vi "更新程序.vi"() -> ()   [LabVIEW 2016, in "数据传输系统.lvlib"]
uses:
  <vilib>/Utility/config.llb/Read Key (String).vi
  <vilib>/Utility/config.llb/Read Key (I32).vi
  <vilib>/Utility/config.llb/NI_LVConfig.lvlib
panel:
  out "软件版本 2":string caption="目标软件版本"
  out "软件版本":string caption="当前软件版本"
  out "下载的文件名":string
  out "目标文件夹名":string
  out "waittime":u8
  out "端口号":i32
  out "IP地址":string
  out "步骤":string
  out "枚举":T1(ring)
  in  "目标路径（使用对话框）":path
  out "下载保存目录":path
  out "更新进度":u8(slide) scale=0.0..100.0
  # "1.先下载更新-------2.关闭主应用-------3.替换应用--------4.打开主应用-----------5.关闭本程序"
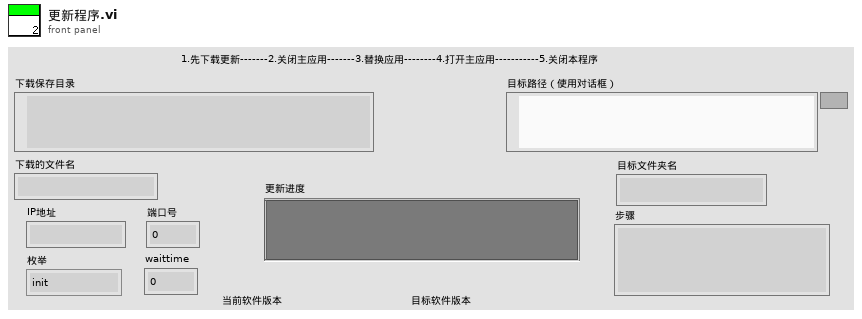
[diagram p1: front panel]
types:
  T1 = enum16{"init", "download", "close", "replace", "open", "over"}
  T2 = enum16{"open", "replace", "create", "open or create", "replace or create", "replace or create with confirmation"}
  T3 = cluster{"网络灯":bool, "接收中":bool, "已接收百分比":u8, "接收成功次数":dbl, "当前步骤":enum16{"init", "receivehead", "receivecontent", "receivesuccess", "over"}, "文件名":string, "error out":errorcluster}
  T4 = typedef "NI_LVConfig.lvlib/Config Data RefNum.ctl" = refnum<k1>
  T5 = enum32{"Bad", "Idle", "Run top level", "Running"}
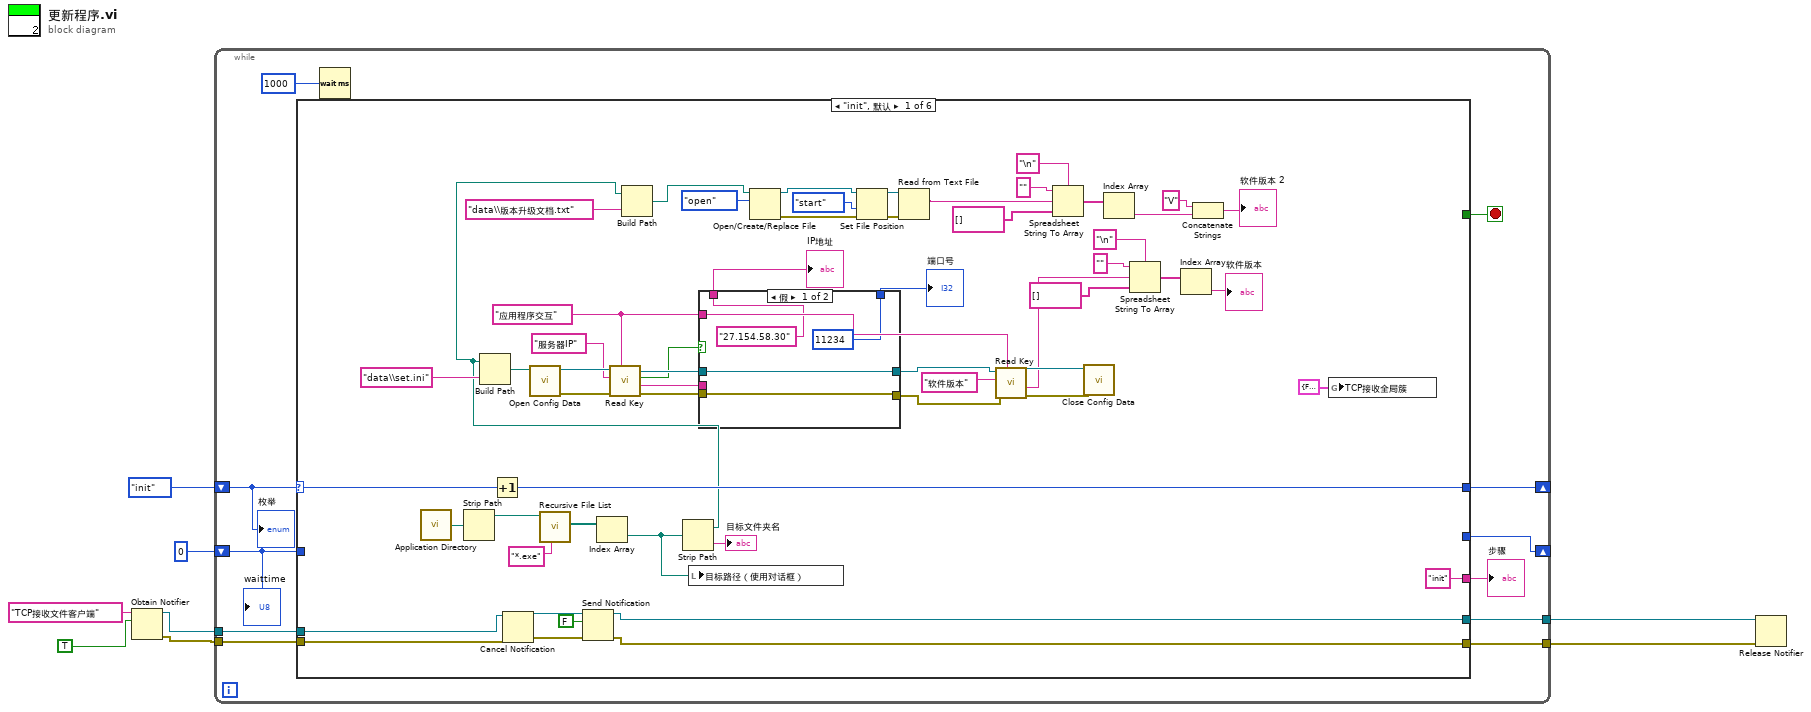
[diagram p0: block diagram]
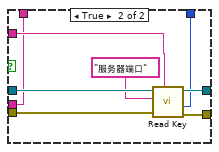
[diagram p2: hidden frame]
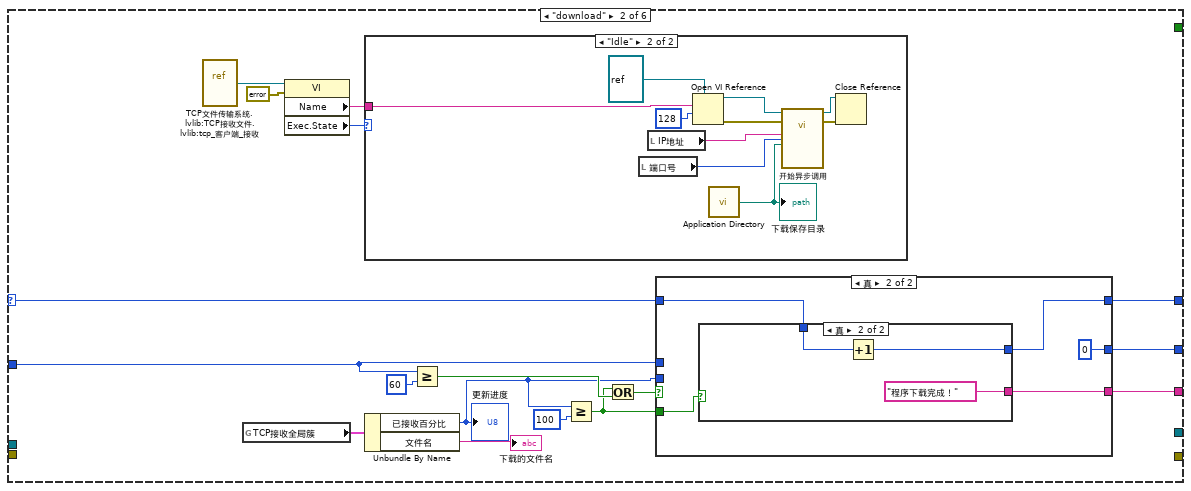
[diagram p3: hidden frame]
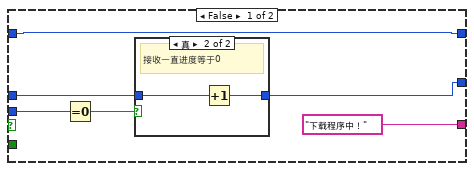
[diagram p5: hidden frame]
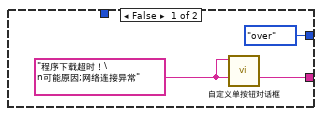
[diagram p7: hidden frame]
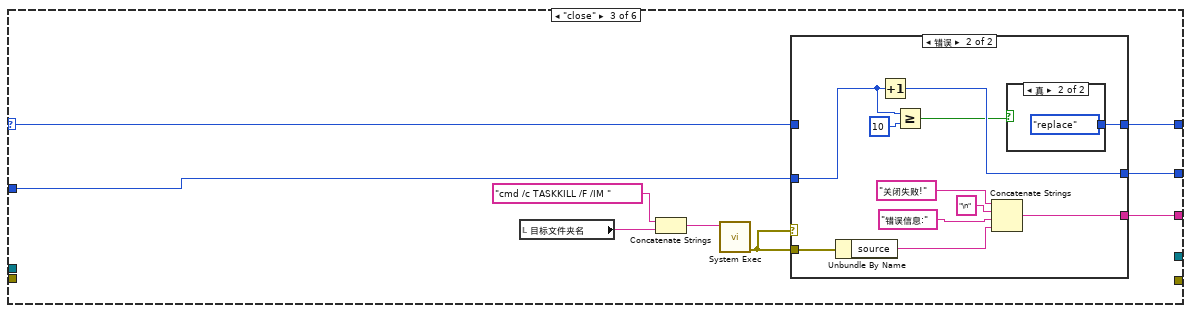
[diagram p8: hidden frame]
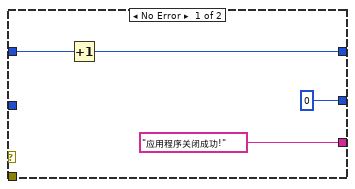
[diagram p9: hidden frame]
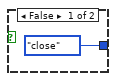
[diagram p10: hidden frame]
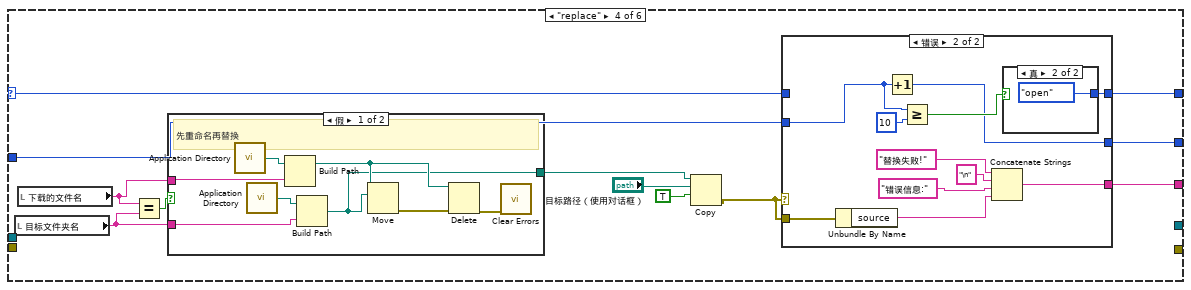
[diagram p11: hidden frame]
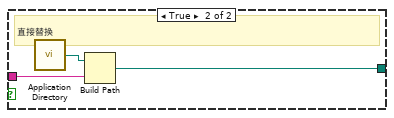
[diagram p12: hidden frame]
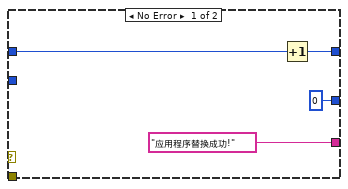
[diagram p13: hidden frame]
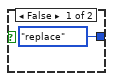
[diagram p14: hidden frame]
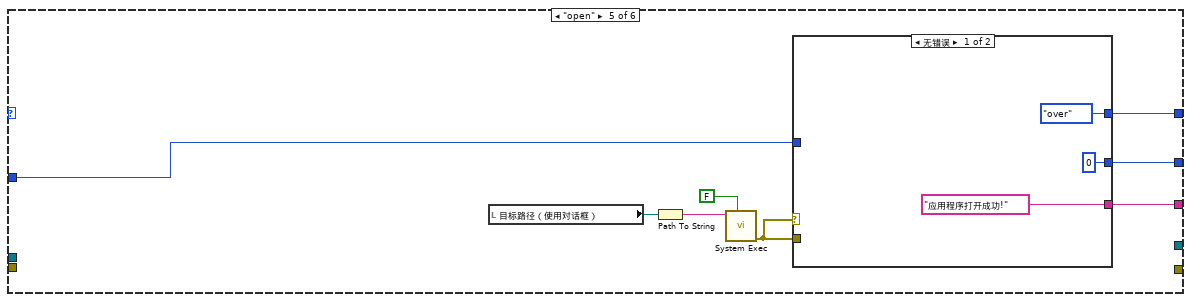
[diagram p15: hidden frame]
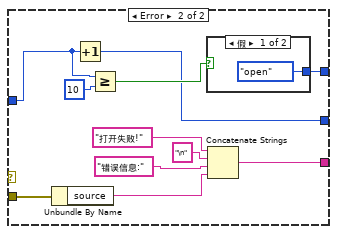
[diagram p16: hidden frame]
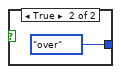
[diagram p17: hidden frame]
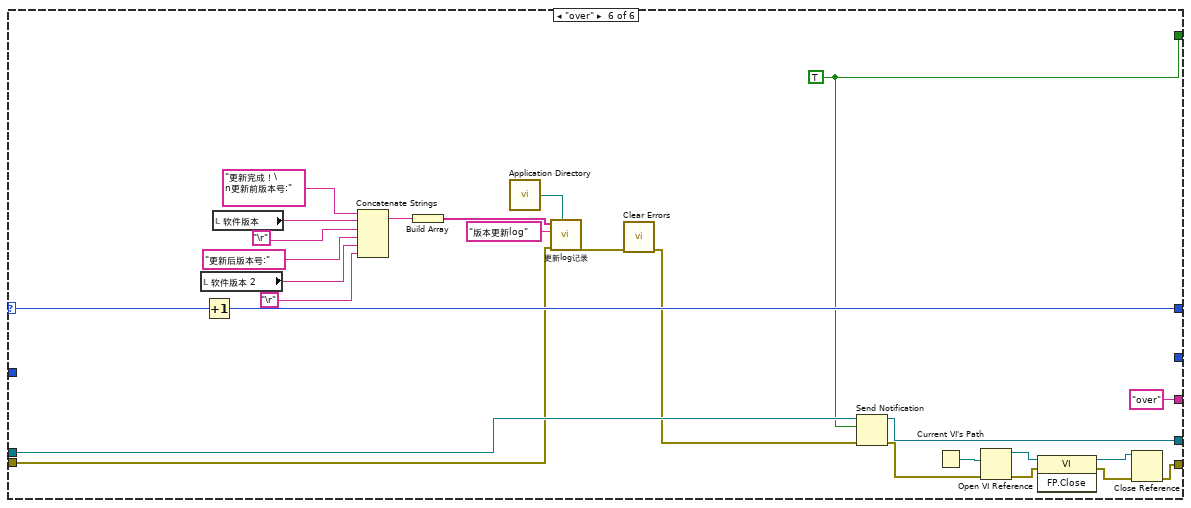
[diagram p18: hidden frame]
diagram:
  n1 = Obtain Notifier(name (unnamed)="TCP接收文件客户端" ("名称（未命名）"), notification data type=TRUE) -> (notifier out=w4:refnum<notifier>, error out=w3:errorcluster)  [unwired: 2 in, 1 out]
  n2 = while {
    shift-right: [w18] -> _
    shift-left: T1."init" -> [w19]
    shift-right: [w13] -> _
    shift-left: u8 0 ("y") -> [w14]
    tunnel: w4 -> [w12]
    tunnel: w3 -> [w11]
    tunnel: [w10] -> w2
    tunnel: [w9] -> w1
    stop <- w17 stop-if-true
    n3 = case shown="\"init\", 默认" w19 {
      selector: w19 -> [w76 w98 w140 w172 _ w250]
      tunnel: [w75 w99 w139 w171 w204 w249] -> w18
      tunnel: [_ _ _ _ _ w245] -> w17
      tunnel: ["init" ("步骤") w95 w138 w170 w203 "over" ("步骤")] -> w15
      tunnel: w14 -> [_ w97 w137 w169 w202 _]
      tunnel: [_ w104 w136 w168 w201 _] -> w13
      tunnel: w12 -> [w73 _ _ _ _ w247]
      tunnel: w11 -> [w72 _ _ _ _ w237]
      tunnel: [w68 _ _ _ _ w246] -> w10
      tunnel: [w67 _ _ _ _ w229] -> w9
      frame "init", Default {
        w47 = "应用程序交互" ("section")
        n4 = call <vilib>:"Application Directory.vi"() -> ("Application Directory"=w64:path)
        n5 = Strip Path(path=w64) -> (stripped path=w60:path)  [unwired: 1 out]
        n6 = Increment(x=w76) -> (x+1=w75:T1)
        n7 = Cancel Notification(0:w73, 3:w72) -> (8:w71:refnum<notifier>, 11:w69:errorcluster)  [unwired: 1 out]
        n8 = call <vilib>:"Recursive File List.vi"("pattern"="*.exe", "Folder Path"=w60) -> ("All Files in Dir"=w62:path[])  [unwired: 5 in, 4 out]
        n9 = Send Notification(notification=FALSE ("通知"), notifier=w71, error in (no error)=w69) -> (notifier out=w68:refnum<notifier>, error out=w67:errorcluster)
        n10 = Index Array(array=w62) -> (element=w65:path)  [unwired: 1 in]
        n11 = Strip Path(path=w65) -> (stripped path=w20:path, name=→"目标文件夹名":string)
        n12 = Build Path(base path=w20, name or relative path="data\\set.ini" ("名称或相对路径")) -> (appended path=w59:path)
        n13 = call <vilib>:"Open Config Data.vi"("configuration file path"=w59) -> ("error out"=w56:errorcluster, "refnum"=w57:T4)  [unwired: 8 in, 1 out]
        n14 = call-poly <vilib>:"Read Key.vi"("section"=w47, "error in (no error)"=w56, "key"="服务器IP" ("section"), "refnum"=w57) -> ("error out"=w46:errorcluster, "value"=w45:string, "found?"=w43:bool, "refnum out"=w55:T4)  [unwired: 4 in]
        n15 = Build Path(base path=w20, name or relative path="data\\版本升级文档.txt" ("名称或相对路径")) -> (appended path=w28:path)
        n16 = local write "目标路径（使用对话框）"(w65) -> ()
        n17 = case shown="假" w43 {
          tunnel: w55 -> [w78 w88]
          tunnel: w46 -> [w77 w87]
          tunnel: [w78 w85] -> w53
          tunnel: [w77 w84] -> w52
          tunnel: [11234 ("value") w83] -> w48
          tunnel: w47 -> [_ w82]
          tunnel: w45 -> [_ w81]
          tunnel: ["27.154.58.30" ("key") w81] -> w44
          frame False {
          }
          frame True {
            n18 = call-poly <vilib>:"Read Key.vi"("section"=w82, "error in (no error)"=w87, "key"="服务器端口" ("section"), "refnum"=w88) -> ("error out"=w84:errorcluster, "value"=w83:i32, "refnum out"=w85:T4)  [unwired: 4 in, 1 out]
          }
        }
        "IP地址" <- w44
        "端口号" <- w48
        n19 = Open/Create/Replace File(file path (use dialog)=w28, operation (0:open)=T2."open" ("操作(0:open)")) -> (refnum out=w23:refnum<file>, error out=w24:errorcluster)  [unwired: 4 in, 1 out]
        n20 = Set File Position(refnum=w23, from (0:start)=enum16{"start", "end", "current"}."start" ("自（0:起始）"), error in=w24) -> (refnum out=w27:refnum<file>, error out=w25:errorcluster)  [unwired: 1 in]
        n21 = Read from Text File(file (use dialog)=w27, error in=w25) -> (text=w35:string)  [unwired: 2 in, 3 out]
        n22 = call-poly <vilib>:"Read Key.vi"("section"=w47, "error in (no error)"=w52, "key"="软件版本", "refnum"=w53) -> ("error out"=w49:errorcluster, "value"=w37:string, "refnum out"=w50:T4)  [unwired: 4 in, 1 out]
        n23 = Spreadsheet String To Array(delimiter (Tab)="\n" ("分隔符(Tab)"), format string="" ("格式字符串"), spreadsheet string=w35, array type (2D Dbl)=string[] []) -> (array=w32:string[])
        n24 = call <vilib>:"Close Config Data.vi"("error in (no error)"=w49, "refnum"=w50) -> ()  [unwired: 8 in, 2 out]
        n25 = Index Array(array=w32) -> (element=w33:string)  [unwired: 1 in]
        n26 = Spreadsheet String To Array(delimiter (Tab)="\n" ("分隔符(Tab)"), format string="" ("格式字符串"), spreadsheet string=w37, array type (2D Dbl)=string[] []) -> (array=w39:string[])
        n27 = Index Array(array=w39) -> (element=→"软件版本":string)  [unwired: 1 in]
        n28 = Concatenate Strings("V" ("字符串"), w33) -> (→"软件版本 2":string)
        n29 = global write "全局变量1.vi" "TCP接收全局簇"(T3 {"网络灯"=FALSE, "接收中"=FALSE, "已接收百分比"=0, "接收成功次数"=0.0, "当前步骤"=enum."init", "文件名"="", "error out"={"status"=FALSE, "code"=0, "source"=""}} ("TCP接收全局簇")) -> ()
      }
      frame "download" {
        n30 = vi-ref "TCP文件传输系统.lvlib:TCP接收文件.lvlib:tcp_客户端_接收.vi"() -> (w90:refnum<vi>)
        n31 = global read "全局变量1.vi" "TCP接收全局簇"() -> (w96:T3)
        n32 = property class="VI"(reference=w90, error in=errorcluster {"status"=FALSE, "code"=0, "source"=""} ("错误输出")) -> ("Name"=w91:string, "Exec.State"=w93:T5)  [unwired: 2 out]
        n33 = case shown="\"Idle\"" w93 {
          tunnel: w91 -> [_ w114]
          frame "Bad", Default {
          }
          frame "Idle" {
            n34 = local read "端口号"() -> (w106:i32)
            n35 = local read "IP地址"() -> (w107:string)
            n36 = Open VI Reference(type specifier VI Refnum (for type only)=refnum<vi> refnum, vi path=w114, options=128 ("选项")) -> (vi reference=w112:refnum<vi>, error out=w110:errorcluster)  [unwired: 3 in]
            n37 = call <vilib>:"Application Directory.vi"() -> ("Application Directory"=w115:path)
            "下载保存目录" <- w115
            n38 = call-by-ref "开始异步调用"(reference=w112, error in=w110, "IP地址"=w107, "端口号"=w106, "储存路径"=w115) -> (reference out=w108:refnum<vi>, error out=w109:errorcluster)  [unwired: 17 in]
            n39 = Close Reference(reference=w108, error in (no error)=w109) -> ()  [unwired: 1 out]
          }
        }
        n40 = Unbundle By Name(w96) -> ("已接收百分比"=w100:u8, "文件名"=→"下载的文件名":string)
        "更新进度" <- w100
        n41 = Greater Or Equal?(x=w97, y=u8 60) -> (x >= y?=w102:bool)
        n42 = Greater Or Equal?(x=w100, y=u8 100) -> (x >= y?=w94:bool)
        n43 = Or(x=w94, y=w102) -> (x .or. y?=w101:bool)
        n44 = case shown="真" w101 {
          tunnel: w97 -> [w121 _]
          tunnel: [w120 u8 0] -> w104
          tunnel: w100 -> [w118 _]
          tunnel: [w117 w125] -> w99
          tunnel: w98 -> [w117 w126]
          tunnel: ["下载程序中！" w127] -> w95
          tunnel: w94 -> [_ w128]
          frame False {
            n45 = Equal To 0?(x=w118) -> (x = 0?=w119:bool)
            n46 = case shown="真" w119 {
              tunnel: w121 -> [w122 w124]
              tunnel: [w122 w123] -> w120
              frame False {
              }
              frame True {
                # "接收一直进度等于0"
                n47 = Increment(x=w124) -> (x+1=w123:u8)
              }
            }
          }
          frame True {
            n48 = case shown="真" w128 {
              tunnel: [w130 "程序下载完成！"] -> w127
              tunnel: w126 -> [_ w133]
              tunnel: [T1."over" w132] -> w125
              frame False {
                w130 = "程序下载超时！\n可能原因;网络连接异常"
                n49 = call "自定义单按钮对话框.vi"("消息"=w130) -> ()  [unwired: 11 in]
              }
              frame True {
                n50 = Increment(x=w133) -> (x+1=w132:T1)
              }
            }
          }
        }
      }
      frame "close" {
        n51 = local read "目标文件夹名"() -> (w135:string)
        n52 = Concatenate Strings("cmd /c TASKKILL /F /IM " ("command line"), w135) -> (w141:string)
        n53 = call <vilib>:"System Exec.vi"("command line"=w141) -> ("error out"=w143:errorcluster)  [unwired: 7 in, 3 out]
        n54 = case shown="错误" w143 {
          tunnel: [w145 w152] -> w139
          tunnel: w143 -> [_ w158]
          tunnel: ["应用程序关闭成功!" ("步骤") w153] -> w138
          tunnel: w140 -> [w146 _]
          tunnel: w137 -> [_ w148]
          tunnel: [u8 0 w150] -> w136
          frame No Error {
            n55 = Increment(x=w146) -> (x+1=w145:T1)
          }
          frame Error {
            n56 = Unbundle By Name(w158) -> ("source"=w157:string)
            n57 = Increment(x=w148) -> (x+1=w150:u8)
            n58 = Greater Or Equal?(x=w148, y=u8 10) -> (x >= y?=w149:bool)
            n59 = Concatenate Strings("关闭失败!" ("消息"), "\n" ("字符串"), "错误信息:" ("字符串"), w157) -> (w153:string)
            n60 = case shown="真" w149 {
              tunnel: [T1."close" T1."replace"] -> w152
              frame False {
              }
              frame True {
              }
            }
          }
        }
      }
      frame "replace" {
        n61 = local read "目标文件夹名"() -> (w164:string)
        n62 = local read "下载的文件名"() -> (w163:string)
        n63 = Equal?(x=w163, y=w164) -> (x = y?=w162:bool)
        n64 = case shown="假" w162 {
          tunnel: w163 -> [w175 w182]
          tunnel: w164 -> [w174 _]
          tunnel: [w173 w181] -> w167
          frame False {
            # "先重命名再替换"
            n65 = call <vilib>:"Application Directory.vi"() -> ("Application Directory"=w176:path)
            n66 = call <vilib>:"Application Directory.vi"() -> ("Application Directory"=w177:path)
            n67 = Build Path(base path=w176, name or relative path=w175) -> (appended path=w178:path)
            n68 = Build Path(base path=w177, name or relative path=w174) -> (appended path=w173:path)
            n69 = Move(source path=w178, 10:w173) -> (error out=w179:errorcluster)  [unwired: 3 in, 2 out]
            n70 = Delete(path (use dialog)=w178, error in=w179) -> (error out=w180:errorcluster)  [unwired: 3 in, 2 out]
            n71 = call <vilib>:"Clear Errors.vi"("error in (no error)"=w180) -> ()  [unwired: 5 in, 2 out]
          }
          frame True {
            # "直接替换"
            n72 = call <vilib>:"Application Directory.vi"() -> ("Application Directory"=w183:path)
            n73 = Build Path(base path=w183, name or relative path=w182) -> (appended path=w181:path)
          }
        }
        n74 = Copy(9:TRUE ("覆盖(F)"), 10:"目标路径（使用对话框）", 11:w167) -> (0:w161:errorcluster)  [unwired: 2 in, 2 out]
        n75 = case shown="错误" w161 {
          tunnel: [w185 w192] -> w171
          tunnel: w161 -> [_ w198]
          tunnel: ["应用程序替换成功!" ("步骤") w193] -> w170
          tunnel: w172 -> [w186 _]
          tunnel: w169 -> [_ w190]
          tunnel: [u8 0 w188] -> w168
          frame No Error {
            n76 = Increment(x=w186) -> (x+1=w185:T1)
          }
          frame Error {
            n77 = Unbundle By Name(w198) -> ("source"=w197:string)
            n78 = Increment(x=w190) -> (x+1=w188:u8)
            n79 = Greater Or Equal?(x=w190, y=u8 10) -> (x >= y?=w189:bool)
            n80 = Concatenate Strings("替换失败!" ("消息"), "\n" ("字符串"), "错误信息:" ("字符串"), w197) -> (w193:string)
            n81 = case shown="真" w189 {
              tunnel: [T1."replace" T1."open"] -> w192
              frame False {
              }
              frame True {
              }
            }
          }
        }
      }
      frame "open" {
        n82 = local read "目标路径（使用对话框）"() -> (w205:path)
        n83 = Path To String(path=w205) -> (string=w208:string)
        n84 = call <vilib>:"System Exec.vi"("wait until completion? (T)"=FALSE, "command line"=w208) -> ("error out"=w206:errorcluster)  [unwired: 6 in, 3 out]
        n85 = case shown="无错误" w206 {
          tunnel: [T1."over" w216] -> w204
          tunnel: w206 -> [_ w222]
          tunnel: ["应用程序打开成功!" ("步骤") w217] -> w203
          tunnel: w202 -> [_ w214]
          tunnel: [u8 0 w212] -> w201
          frame No Error {
          }
          frame Error {
            n86 = Unbundle By Name(w222) -> ("source"=w221:string)
            n87 = Increment(x=w214) -> (x+1=w212:u8)
            n88 = Greater Or Equal?(x=w214, y=u8 10) -> (x >= y?=w213:bool)
            n89 = case shown="假" w213 {
              tunnel: [T1."open" T1."over"] -> w216
              frame False {
              }
              frame True {
              }
            }
            n90 = Concatenate Strings("打开失败!" ("消息"), "\n" ("字符串"), "错误信息:" ("字符串"), w221) -> (w217:string)
          }
        }
      }
      frame "over" {
        w245 = TRUE
        n91 = local read "软件版本 2"() -> (w226:string)
        n92 = Increment(x=w250) -> (x+1=w249:T1)
        n93 = local read "软件版本"() -> (w228:string)
        n94 = Concatenate Strings("更新完成！\n更新前版本号:" ("字符串"), w228, "\r", "更新后版本号:", w226, "\r") -> (w243:string)
        n95 = Build Array(w243) -> (w242:string[])
        n96 = call <vilib>:"Application Directory.vi"() -> ("Application Directory"=w240:path)
        n97 = call "更新log记录.vi"("路径"=w240, "错误输入（无错误）"=w237, "logname"="版本更新log", "数组"=w242) -> ("错误输出"=w238:errorcluster)  [unwired: 7 in]
        n98 = call <vilib>:"Clear Errors.vi"("error in (no error)"=w238) -> ("error out"=w236:errorcluster)  [unwired: 5 in, 1 out]
        n99 = Send Notification(notification=w245, notifier=w247, error in (no error)=w236) -> (notifier out=w246:refnum<notifier>, error out=w232:errorcluster)
        n100 = Current VI's Path() -> (path=w234:path)
        n101 = Open VI Reference(vi path=w234, error in (no error)=w232) -> (vi reference=w233:refnum<vi>, error out=w235:errorcluster)  [unwired: 4 in]
        n102 = invoke class="VI" method="FP.Close"(reference=w233, error in=w235) -> (reference out=w230:refnum<vi>, error out=w231:errorcluster)  [unwired: 1 in, 1 out]
        n103 = Close Reference(reference=w230, error in (no error)=w231) -> (error out=w229:errorcluster)
      }
    }
    "步骤" <- w15
    n104 = Wait (ms)(milliseconds to wait=u32 1000 ("等待时间（毫秒）")) -> ()  [unwired: 1 out]
    "枚举" <- w19
    "waittime" <- w14
  }
  n105 = Release Notifier(notifier=w2, error in (no error)=w1) -> ()  [unwired: 1 in, 3 out]
